vi "Initialize MeasurementLink Session.vi"(7 "remote connection options":T2, 8 "error in":errorcluster, 9 "initialize session behavior":T1, 10 "resource name":string, 11 "instrument in":refnum<class "Instrument.lvclass">) -> (0 "error out":errorcluster, 2 "session out":variant, 3 "instrument out":refnum<class "Instrument.lvclass">)   [LabVIEW 2020, in "MeasurementLink 34401.lvlib" / "Instrument.lvclass"]
uses:
  Instrument.lvclass
  Instrument.lvclass/Instrument.ctl
  <vilib>/MeasurementLink/MeasurementLink Measurement Server/Helpers/Error Strings Global Internal.vi
  <instrlib>/Agilent 34401/Agilent 34401.lvlib
  <vilib>/MeasurementLink/MeasurementLink Instrument/IInstrument/Initialize Session Behavior.ctl
  <vilib>/MeasurementLink/MeasurementLink Instrument/IInstrument/IInstrument.lvclass
  <vilib>/MeasurementLink/MeasurementLink Instrument/IInstrument/Remote Connection Options.ctl
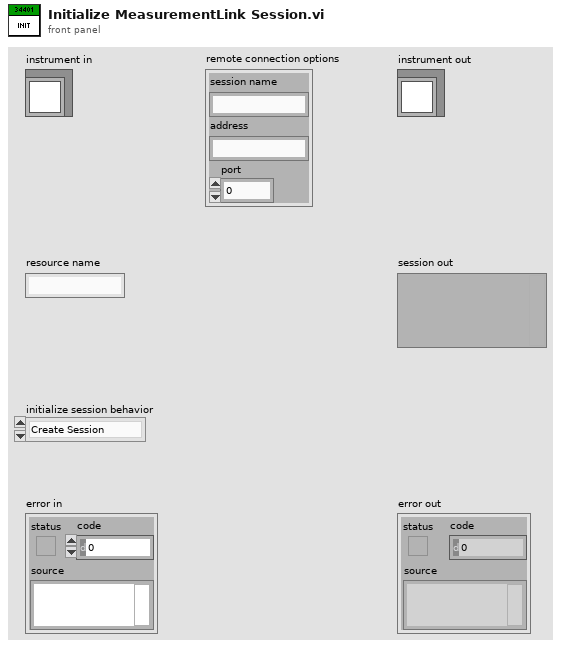
[diagram p1: front panel]
types:
  T1 = typedef "MeasurementLink Instrument.lvlib/IInstrument.lvclass/Initialize Session Behavior.ctl" = enum16{"Create Session", "Attach Session"}
  T2 = typedef "MeasurementLink Instrument.lvlib/IInstrument.lvclass/Remote Connection Options.ctl" = cluster{"session name":string, "address":string, "port":u32}
  T3 = cluster{"Baud Rate":u32, "Parity":u16, "Data Bits":u16}
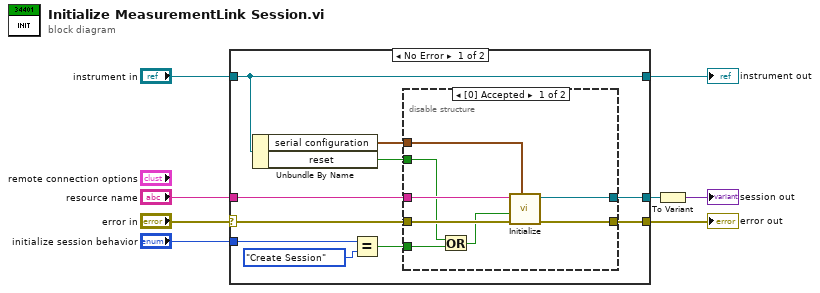
[diagram p0: block diagram]
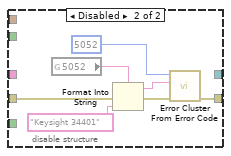
[diagram p2: hidden frame]
diagram:
  n1 = case shown="No Error" "error in" {
    selector: "error in" -> [w17 w34]
    tunnel: [w16 w34] -> w7
    tunnel: "instrument in" -> [w14 w35]
    tunnel: [w14 w35] -> w5
    tunnel: "initialize session behavior" -> [w12 _]
    tunnel: "resource name" -> [w15 _]
    tunnel: [w18 _] -> w2
    frame No Error {
      n2 = Unbundle By Name(w14) -> ("serial configuration"=w13:T3, "reset"=w9:bool)
      n3 = Equal?(x=w12, y=Initialize_Session_Behavior."Create Session" ("initialize session behavior")) -> (x = y?=w10:bool)
      n4 = disable-structure shown="[0] Accepted" {
        disable-tunnel: [w26 _] -> w18
        disable-tunnel: w17 -> [w25 w27]
        disable-tunnel: [w24 w28] -> w16
        disable-tunnel: w15 -> [w23 _]
        disable-tunnel: w13 -> [w20 _]
        disable-tunnel: w10 -> [w22 _]
        disable-tunnel: w9 -> [w19 _]
        frame Enabled {
          n5 = Or(x=w19, y=w22) -> (x .or. y?=w21:bool)
          n6 = call <instrlib>:"Initialize.vi"("Serial Configuration"=w20, "error in (no error)"=w25, "Reset (True)"=w21, "VISA resource name"=w23) -> ("error out"=w24:errorcluster, "VISA resource name out"=w26:refnum<visa-resource-name>)  [unwired: 6 in]
        }
        frame Disabled {
          n7 = global read "Error Strings Global Internal.vi" "5052"() -> (w32:string)
          n8 = Format Into String(format string=w32, error in=w27, "Keysight 34401") -> (resulting string=w29:string, error out=w30:errorcluster)  [unwired: 1 in]
          n9 = call <vilib>:"Error Cluster From Error Code.vi"("error in (no error)"=w30, "error message (\"\")"=w29, "error code (0)"=5052) -> ("error out"=w28:errorcluster)  [unwired: 6 in]
        }
      }
    }
    frame Error {
    }
  }
  "error out" <- w7
  "instrument out" <- w5
  n10 = To Variant(anything=w2) -> (Variant=→"session out":variant)
